vi "Connect Initialize APIs.vi"(5 "sub vis":refnum<vi>[](array[refnum]), 11 "error in":errorcluster) -> (15 "error out":errorcluster)   [LabVIEW 2021, in "Converter.lvlib"]
uses:
  Converter.lvlib
  Converter Reusables/Converter Reusables.lvlib
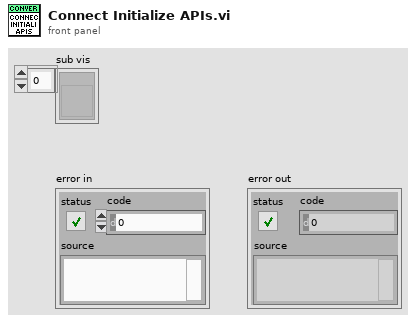
[diagram p1: front panel]
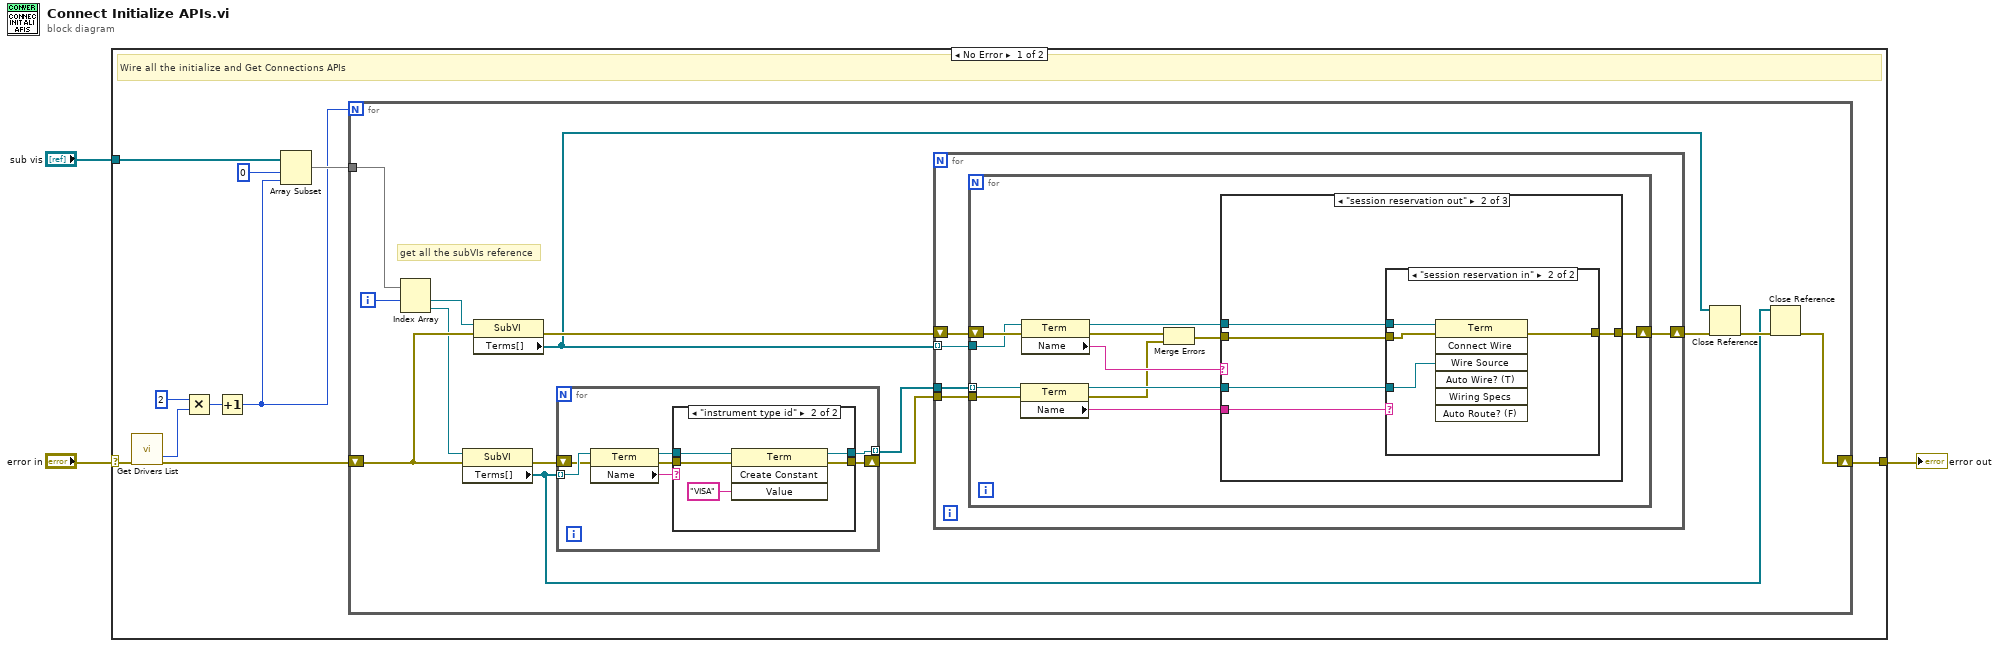
[diagram p0: block diagram]
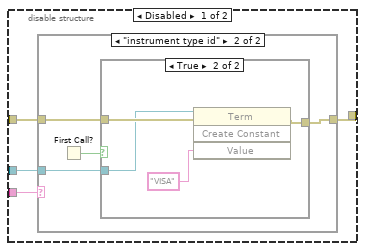
[diagram p3: hidden frame]
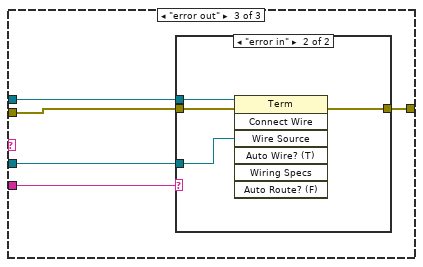
[diagram p7: hidden frame]
diagram:
  n1 = case shown="No Error" "error in" {
    selector: "error in" -> [w12 w98]
    tunnel: "sub vis" -> [w13 _]
    tunnel: [w8 w98] -> w1
    frame No Error {
      # "Wire all the initialize and Get Connections APIs"
      n2 = call "Get Drivers List.vi"("error in"=w12) -> ("removed duplicates size"=w7:i32, "error out"=w9:errorcluster)  [unwired: 9 in, 4 out]
      n3 = Multiply(x=2, y=w7) -> (x*y=w5:i32)
      n4 = Increment(x=w5) -> (x+1=w4:i32)
      n5 = Array Subset(array=w13, index=0, length=w4) -> (w10:refnum<vi>[])
      n6 = for {
        N: w4 -> [_]
        tunnel: w10 -> [w26]
        shift-right: [w24] -> w8
        shift-left: w9 -> [w25]
        i -> [w27]
        # "get all the subVIs reference"
        n7 = Index Array(array=w26, index #1=w27) -> (element #1=w23:refnum<vi>, element #2=w22:refnum<vi>)  [unwired: 1 in]
        n8 = property class="SubVI"(reference=w22, error in=w25) -> (error out=w17:errorcluster, "Terms[]"=w16:refnum<vi>[])  [unwired: 1 out]
        n9 = property class="SubVI"(reference=w23, error in=w25) -> (error out=w21:errorcluster, "Terms[]"=w19:refnum<vi>[])  [unwired: 1 out]
        n10 = for {
          tunnel: w16 -> [w90] mode=indexing
          tunnel: [w84] -> w14 mode=indexing
          shift-right: [w87] -> w15
          shift-left: w17 -> [w89]
          n11 = property class="Term"(reference=w90, error in=w89) -> (reference out=w85:refnum<vi>, error out=w88:errorcluster, "Name"=w86:string)
          n12 = case shown="\"instrument type id\"" w86 {
            tunnel: w88 -> [w92 w97]
            tunnel: [w92 w96] -> w87
            tunnel: w85 -> [w91 w95]
            tunnel: [w91 w94] -> w84
            frame Default {
            }
            frame "instrument type id" {
              n13 = invoke class="Term" method="Create Constant"(reference=w95, error in=w97, "Value"="VISA") -> (reference out=w94:refnum<vi>, error out=w96:errorcluster)  [unwired: 1 in, 2 out]
            }
          }
        }
        n14 = for {
          tunnel: w19 -> [w31] mode=indexing
          tunnel: w15 -> [w30]
          shift-right: [w29] -> w20
          shift-left: w21 -> [w32]
          tunnel: w14 -> [w28]
          n15 = for {
            tunnel: w31 -> [w43]
            tunnel: w30 -> [w42]
            shift-right: [w34] -> w29
            shift-left: w32 -> [w44]
            tunnel: w28 -> [w33] mode=indexing
            n16 = property class="Term"(reference=w33, error in=w42) -> (reference out=w37:refnum<vi>, error out=w35:errorcluster, "Name"=w40:string)
            n17 = property class="Term"(reference=w43, error in=w44) -> (reference out=w38:refnum<vi>, error out=w39:errorcluster, "Name"=w41:string)
            n18 = Merge Errors(w39, w35) -> (w36:errorcluster)
            n19 = case shown="\"session reservation out\"" w41 {
              tunnel: w40 -> [w48 w68 w78]
              tunnel: w36 -> [w47 w67 w77]
              tunnel: w38 -> [_ w65 w76]
              tunnel: w37 -> [w46 w64 w75]
              tunnel: [w45 w66 w74] -> w34
              frame Default {
                n20 = disable-structure shown="Enabled" {
                  disable-tunnel: w48 -> [w52 _]
                  disable-tunnel: w47 -> [w51 w63]
                  disable-tunnel: w46 -> [w50 _]
                  disable-tunnel: [w49 w63] -> w45
                  frame Disabled {
                    n21 = case shown="\"instrument type id\"" w52 {
                      tunnel: w51 -> [w53 w56]
                      tunnel: w50 -> [_ w55]
                      tunnel: [w53 w54] -> w49
                      frame Default {
                      }
                      frame "instrument type id" {
                        n22 = First Call?() -> (First Call?: T/F=w57:bool)
                        n23 = case shown="True" w57 {
                          tunnel: w56 -> [w58 w62]
                          tunnel: w55 -> [_ w61]
                          tunnel: [w58 w59] -> w54
                          frame False {
                          }
                          frame True {
                            n24 = invoke class="Term" method="Create Constant"(reference=w61, error in=w62, "Value"="VISA") -> (error out=w59:errorcluster)  [unwired: 1 in, 3 out]
                          }
                        }
                      }
                    }
                  }
                  frame Enabled {
                  }
                }
              }
              frame "session reservation out" {
                n25 = case shown="\"session reservation in\"" w68 {
                  tunnel: w67 -> [w69 w72]
                  tunnel: [w69 w70] -> w66
                  tunnel: w65 -> [_ w73]
                  tunnel: w64 -> [_ w71]
                  frame Default {
                  }
                  frame "session reservation in" {
                    n26 = invoke class="Term" method="Connect Wire"(reference=w73, error in=w72, "Wire Source"=w71) -> (error out=w70:errorcluster)  [unwired: 4 in, 6 out]
                  }
                }
              }
              frame "error out" {
                n27 = case shown="\"error in\"" w78 {
                  tunnel: w77 -> [w79 w81]
                  tunnel: w76 -> [_ w83]
                  tunnel: w75 -> [_ w82]
                  tunnel: [w79 w80] -> w74
                  frame Default {
                  }
                  frame "error in" {
                    n28 = invoke class="Term" method="Connect Wire"(reference=w83, error in=w81, "Wire Source"=w82) -> (error out=w80:errorcluster)  [unwired: 4 in, 6 out]
                  }
                }
              }
            }
          }
        }
        n29 = Close Reference(reference=w19, error in (no error)=w20) -> (error out=w18:errorcluster)
        n30 = Close Reference(reference=w16, error in (no error)=w18) -> (error out=w24:errorcluster)
      }
    }
    frame Error {
    }
  }
  "error out" <- w1
